vi "GraphFacade.vi"(0 "Data In":T5 {"Settings"."Time" format="%<%H:%M\n%d/%m/%y>T"}, 2 "Display State In":T3, 3 "Container State":T4) -> (6 "Data Out":T5 {"Settings"."Time" format="%<%H:%M\n%d/%m/%y>T"}, 7 "Display State Out":T3, 8 "Action":T2)   [LabVIEW 2014, in "SpectralView.xctl"]
uses:
  <userlib>/CurtinCode/Graphctrl/SpectralView.xctl
  <userlib>/CurtinCode/Graphctrl/GraphData.ctl
  <userlib>/CurtinCode/DataControl.ctl
  <userlib>/CurtinCode/SettingsControl.ctl
  <vilib>/_xctls/Container State.ctl
  <userlib>/CurtinCode/Graphctrl/GraphState.ctl
  <vilib>/_xctls/Action.ctl
  <vilib>/_xctls/XControlSupport.lvlib
panel:
  in  "Cursor Data":string[][](table)
  out "Magnitude":T1(graph)=[{0.0, "df"=1.46484375, "Power Spectrum (V^2 rms)"=array[16384 elements]}, {0.0, "df"=1.46484375, "Power Spectrum (V^2 rms)"=array[6612 elements]}]
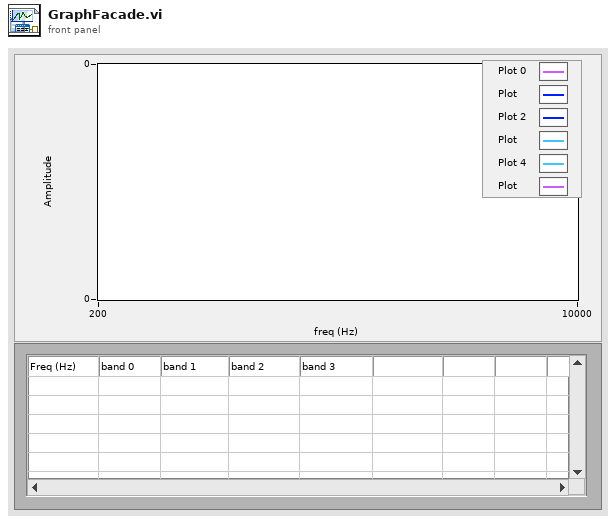
[diagram p1: front panel]
types:
  T1 = cluster{dbl, "df":dbl, "Power Spectrum (V^2 rms)":dbl[]}[]
  T2 = typedef "XControlSupport.lvlib/Action.ctl" = cluster{"Data Changed?":bool, "State Changed?":bool, "Action Name":string}
  T3 = typedef "SpectralView.xctl/GraphState.ctl" = cluster{"Numeric":dbl}
  T4 = typedef "XControlSupport.lvlib/Container State.ctl" = cluster{"Indicator?":bool, "Run Mode?":bool, " Refnum":refnum<vi>}
  T5 = typedef "SpectralView.xctl/GraphData.ctl" = T6[]
  T6 = typedef "DataControl.ctl" = cluster{"Settings":T7, "Data":cluster{i32, dbl, "data":dbl[]}[], "Plot type":enum16{"Linear", "log"}}
  T7 = typedef "SettingsControl.ctl" = cluster{"Data Path":path, "Time":timestamp, "Sampling Rate (Hz)":u16, "Device":u16, "pre-trigger (sec)":dbl, "length of sample (sec)":dbl, "trigger value (V)":dbl, "Labels":string[], "Cutoffs (V)":dbl[], "Freq Bands":dbl[]}
  T8 = cluster{"Name":string, "Color":u32, "Style":u8, "Point Style":u8, "Name Visible":bool, "Allow Drag":bool, "Cursor Mode":u32, "Plot":i32, "Index":i32, "Position":cluster{"X":dbl, "Y":dbl}, "X Scale":u32, "Y Scale":u32, "Watch Plots":i32[], "Watch All Plots":bool, "Plot Area":i32, "Label Offset":cluster{"X":dbl, "Y":dbl}}
  T9 = typedef "LVCursorListTypeDef.ctl" = cluster{"Name":string, "Color":u32, "Style":u8, "Point Style":u8, "Name Visible":bool, "Allow Drag":bool, "Cursor Mode":u32, "Plot":i32, "Index":i32, "Position":cluster{"X":dbl, "Y":dbl}, "X Scale":u32, "Y Scale":u32, "Watch Plots":i32[], "Watch All Plots":bool, "Plot Area":i32, "Label Offset":cluster{"X":dbl, "Y":dbl}}[]
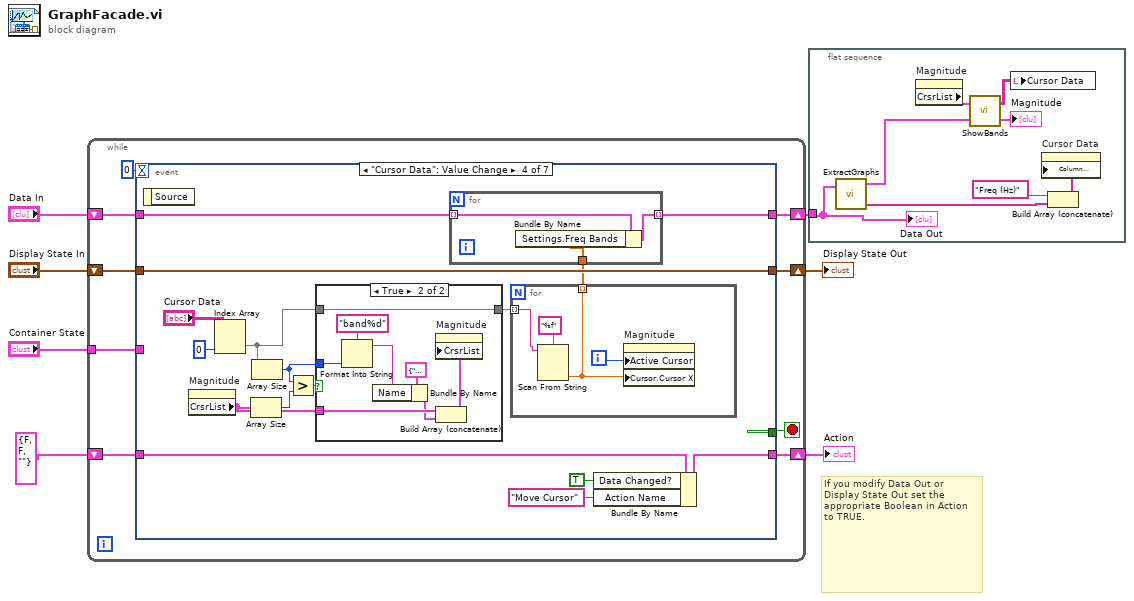
[diagram p0: block diagram]
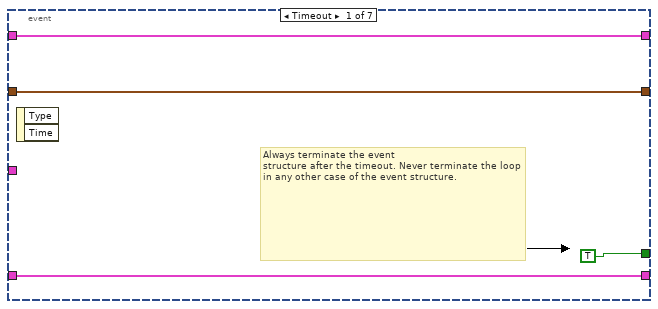
[diagram p2: hidden frame]
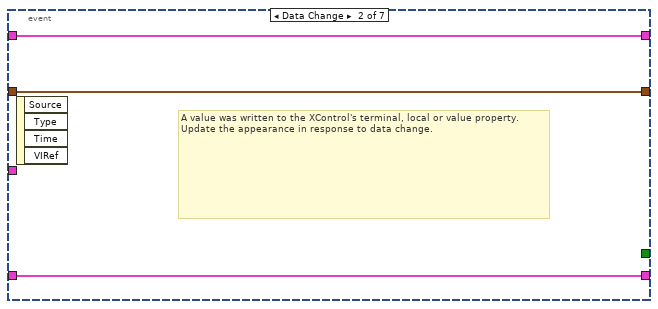
[diagram p3: hidden frame]
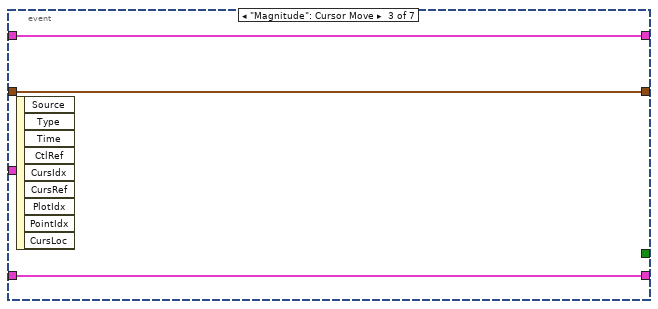
[diagram p4: hidden frame]
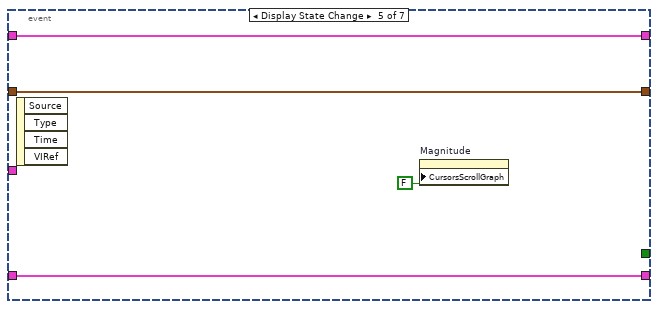
[diagram p6: hidden frame]
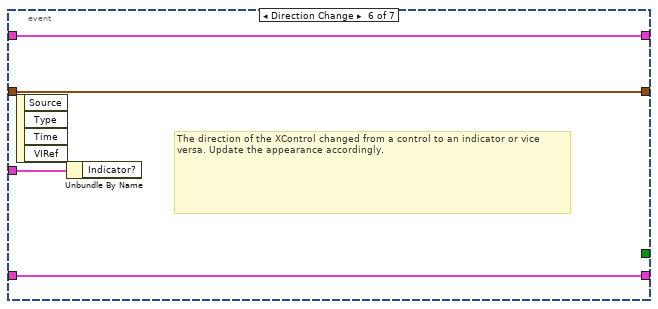
[diagram p7: hidden frame]
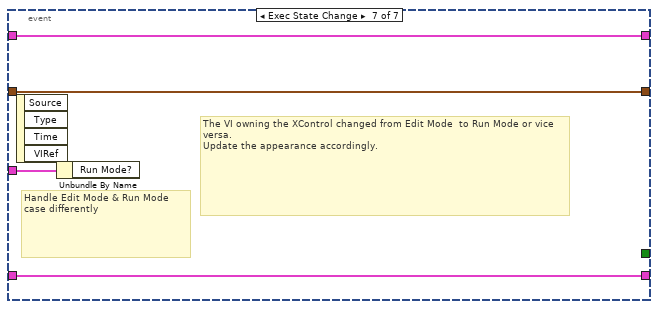
[diagram p8: hidden frame]
diagram:
  # "If you modify Data Out or\nDisplay State Out set the\nappropriate Boolean in Action\nto TRUE."
  n1 = while {
    shift-right: [w15] -> w5
    shift-left: "Display State In" -> [w16]
    tunnel: "Container State" -> [w12]
    shift-right: [w10] -> w1
    shift-left: "Data In" -> [w11]
    shift-right: [w8] -> w3
    shift-left: T2 {"Data Changed?"=FALSE, "State Changed?"=FALSE, "Action Name"=""} ("Action") -> [w9]
    stop <- w14 stop-if-true
    n2 = event shown="[3] \"Cursor Data\": Value Change" {
      selector: _ -> [_ _ _ _ _ _ _]
      dyn-events: _ -> [_ _ _ _ _ _ _]
      timeout: 0 -> [_ _ _ _ _ _ _]
      tunnel: w16 -> [w18 w22 w26 w42 w62 w65 w69]
      tunnel: [w18 w22 w26 w42 w62 w65 w69] -> w15
      tunnel: [TRUE _ _ _ _ _ _] -> w14
      tunnel: w12 -> [_ _ _ _ _ w66 w70]
      tunnel: w11 -> [w17 w23 w24 w29 w61 w64 w68]
      tunnel: [w17 w23 w24 w27 w61 w64 w68] -> w10
      tunnel: [w19 w21 w25 w32 w60 w63 w67] -> w8
      tunnel: w9 -> [w19 w21 w25 w33 w60 w63 w67]
      event Timeout {
        # "Always terminate the event\nstructure after the timeout. Never terminate the loop in any other case of the event structure."
        n3 = event-data() -> ()  [unwired: 1 in, 2 out]
      }
      event Data Change {
        # "A value was written to the XControl's terminal, local or value property.\nUpdate the appearance in response to data change."
        n4 = event-data() -> ()  [unwired: 1 in, 4 out]
      }
      event "Magnitude": Cursor Move {
        n5 = event-data() -> ()  [unwired: 1 in, 9 out]
      }
      event "Cursor Data": Value Change {
        n6 = event-data() -> ()  [unwired: 1 in, 1 out]
        n7 = property on="Magnitude" class="WFGraph (strict)"() -> ("CrsrList"=w37:T9)  [unwired: 2 in, 2 out]
        n8 = Index Array(array="Cursor Data", index (col)=0 ("disabled index (col)")) -> (element=w34:string[])  [unwired: 1 in]
        n9 = Array Size(array=w37) -> (size(s)=w39:i32)
        n10 = Array Size(array=w34) -> (size(s)=w36:i32)
        n11 = Greater?(x=w36, y=w39) -> (0:w38:bool)
        n12 = case shown="True" w38 {
          tunnel: w37 -> [_ w54]
          tunnel: w36 -> [_ w50]
          tunnel: [w46 w47] -> w35
          tunnel: w34 -> [w46 w47]
          frame False {
          }
          frame True {
            n13 = Format Into String(format string="band%d", w50) -> (resulting string=w48:string)  [unwired: 2 in, 1 out]
            n14 = Bundle By Name(cluster=T8 {"Name"="", "Color"=0, "Style"=0, "Point Style"=0, "Name Visible"=FALSE, "Allow Drag"=FALSE, "Cursor Mode"=0, "Plot"=0, "Index"=0, "Position"={"X"=0.0, "Y"=0.0}, "X Scale"=0, "Y Scale"=0, "Watch Plots"=[], "Watch All Plots"=FALSE, "Plot Area"=0, "Label Offset"={"X"=0.0, "Y"=0.0}}, "Name"=w48) -> (w51:T8)
            n15 = Build Array (concatenate)(w54, w51) -> (w53:T9)
            n16 = property on="Magnitude" class="WFGraph (strict)"("CrsrList"=w53) -> ()  [unwired: 2 in, 2 out]
          }
        }
        n17 = for {
          tunnel: w35 -> [w56] mode=indexing
          tunnel: [w55] -> w28 mode=indexing
          i -> [w57]
          n18 = Scan From String(format string="%f", input string=w56) -> (output 1=w55:dbl)  [unwired: 3 in, 3 out]
          n19 = property on="Magnitude" class="WFGraph (strict)"("Active Cursor"=w57, "Cursor.Cursor X"=w55) -> ()  [unwired: 2 in, 2 out]
        }
        n20 = for {
          tunnel: w29 -> [w45] mode=indexing
          tunnel: w28 -> [w44]
          tunnel: [w43] -> w27 mode=indexing
          n21 = Bundle By Name(cluster=w45, "Settings.Freq Bands"=w44) -> (w43:T6)
        }
        n22 = Bundle By Name(cluster=w33, "Data Changed?"=TRUE, "Action Name"="Move Cursor") -> (w32:T2)
      }
      event Display State Change {
        n23 = event-data() -> ()  [unwired: 1 in, 4 out]
        n24 = property on="Magnitude" class="WFGraph (strict)"("CursorsScrollGraph"=FALSE ("Cursors Scroll Graph")) -> ()  [unwired: 2 in, 2 out]
      }
      event Direction Change {
        # "The direction of the XControl changed from a control to an indicator or vice versa. Update the appearance accordingly."
        n25 = event-data() -> ()  [unwired: 1 in, 4 out]
        n26 = Unbundle By Name(w66) -> ()  [unwired: 1 out]
      }
      event Exec State Change {
        # "The VI owning the XControl changed from Edit Mode  to Run Mode or vice versa.\nUpdate the appearance accordingly."
        # "Handle Edit Mode & Run Mode\ncase differently"
        n27 = event-data() -> ()  [unwired: 1 in, 4 out]
        n28 = Unbundle By Name(w70) -> ()  [unwired: 1 out]
      }
    }
  }
  "Display State Out" <- w5
  "Action" <- w3
  n29 = flat-sequence {
    tunnel: w1 -> [w73]
    frame #0 {
      n30 = call <userlib>:"ExtractGraphs.vi"("Spectra Out"=w73) -> ("Mag"=w72:cluster{i32, dbl, "data":dbl[]}[], "FileNames"=w71:string[])  [unwired: 2 out]
      n31 = property on="Magnitude" class="WFGraph (strict)"() -> ("CrsrList"=w78:T9)  [unwired: 2 in, 2 out]
      n32 = call <userlib>:"ShowBands.vi"("Magnitude"=w72, "CrsrList"=w78) -> ("Normalized FFT"=→"Magnitude":T1, "Cursor Data"=w76:string[][])
      n33 = local write "Cursor Data"(w76) -> ()
      n34 = Build Array (concatenate)("Freq (Hz)" ("format string"), w71) -> (w74:string[])
      n35 = property on="Cursor Data" class="Tbl (strict)"("Column Headers[]"=w74) -> ()  [unwired: 2 in, 2 out]
      "Data Out" <- w73
    }
  }
